vi "Set Initialization Data - Modbus PLC.vi"(8 "error in":errorcluster, 11 "gui in":refnum<class "gui.lvclass">) -> (0 "error out":errorcluster, 3 "gui out":refnum<class "gui.lvclass">)   [LabVIEW 2023, in "GUI.lvlib" / "gui.lvclass"]
doc: "In this VI you can set the initialization data of a statically-linked subWorker."
uses:
  gui.lvclass
  Modbus PLC/Modbus PLC/Initialization Data.ctl
  <vilib>/addons/_Workers/Library/Case Label.ctl
  gui.lvclass/gui.ctl
  Modbus PLC/Modbus PLC/Modbus PLC.lvclass
  <vilib>/addons/_Workers/Library/Workers.lvlib
  Workers Hardware/Workers/Base Classes/Base Hardware/Settings.ctl
  Workers Hardware/Workers/Base Classes/Base Hardware/Base Hardware.lvclass
  Workers Hardware/Workers/Base Classes/Base Hardware/Response Cases.ctl
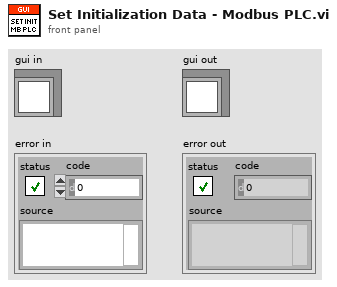
[diagram p1: front panel]
types:
  T1 = typedef "Modbus PLC.lvlib/Modbus PLC.lvclass/Initialization Data.ctl" = cluster{"Response Cases":T2, "Settings":T4}
  T2 = typedef "Abstract Hardware.lvlib/Base Hardware.lvclass/Response Cases.ctl" = cluster{"Placeholder - Can be deleted":string, "Get Data":T3, "Get Init Result":T3}
  T3 = typedef "Workers.lvlib/Case Label.ctl" = string
  T4 = typedef "Abstract Hardware.lvlib/Base Hardware.lvclass/Settings.ctl" = cluster{"Polling Period, ms":i64}
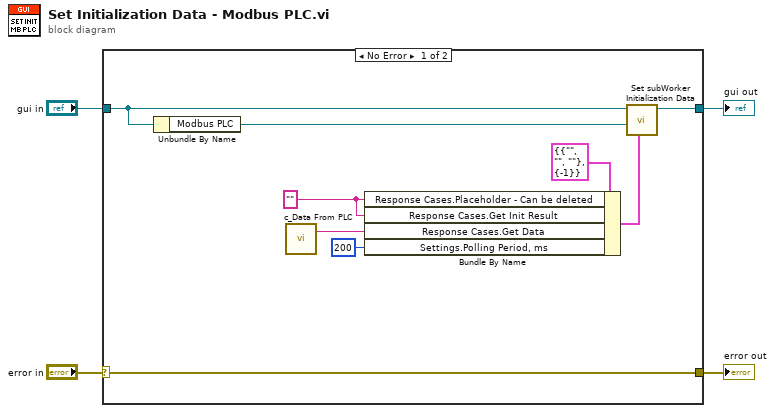
[diagram p0: block diagram]
diagram:
  n1 = case shown="No Error" "error in" {
    selector: "error in" -> [w13 w15]
    tunnel: [w13 w15] -> w3
    tunnel: [w11 w14] -> w2
    tunnel: "gui in" -> [w10 w14]
    frame No Error {
      w7 = "" ("Placeholder")
      n2 = Unbundle By Name(w10) -> ("Modbus PLC"=w12:refnum<class "Modbus PLC.lvclass">)
      n3 = call "c_Data From PLC.vi"() -> ("Case Label"=w6:T3)  [unwired: 1 in]
      n4 = Bundle By Name(cluster=T1 {"Response Cases"={"Placeholder - Can be deleted"="", "Get Data"="", "Get Init Result"=""}, "Settings"={"Polling Period, ms"=-1}} ("Initialization Data"), "Response Cases.Placeholder - Can be deleted"=w7, "Response Cases.Get Init Result"=w7, "Response Cases.Get Data"=w6, "Settings.Polling Period, ms"=i64 200) -> (w8:T1)
      n5 = call-dynamic "Set subWorker Initialization Data.vi"("Initialization Data"=w8, "subWorker"=w12, "Worker"=w10) -> ("Worker out"=w11:refnum<class "gui.lvclass">)  [unwired: 8 in]
    }
    frame Error {
    }
  }
  "error out" <- w3
  "gui out" <- w2
